vi "Transfer State 3 test.vi"() -> ()   [LabVIEW 2019]
panel:
  out "s? t:f":dbl
  in  "x":bool
  in  "Reset":bool
  in  "Transfer Forward Slow":dbl
  in  "Transfer Rev slow":dbl
  in  "Transfer Rev Fast":dbl
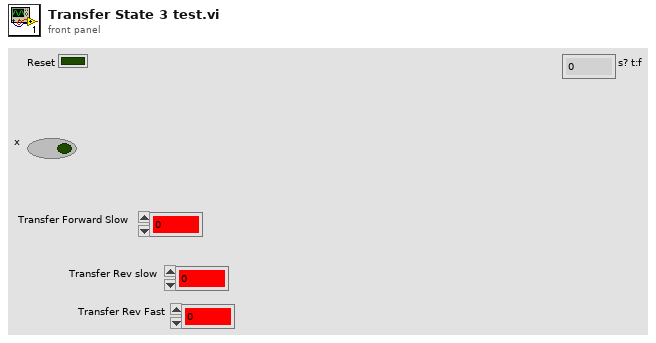
[diagram p1: front panel]
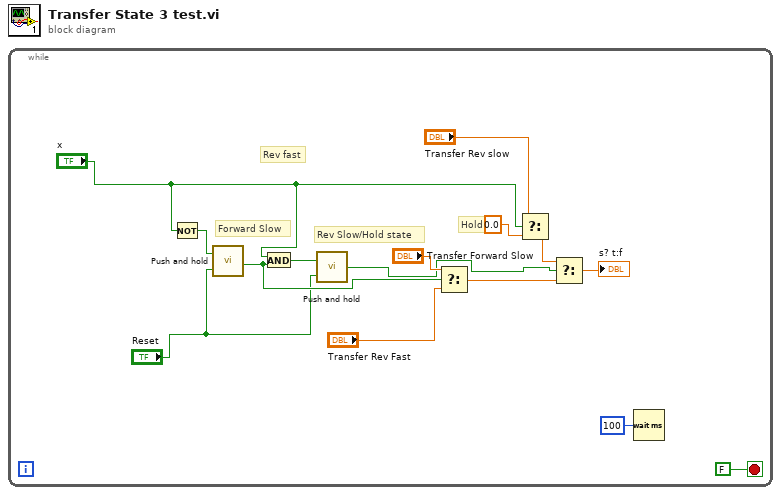
[diagram p0: block diagram]
diagram:
  n1 = while {
    stop <- FALSE stop-if-true
    # "Hold"
    # "Rev Slow/Hold state"
    # "Forward Slow"
    # "Rev fast"
    n2 = Not(x="x") -> (.not. x?=w15:bool)
    n3 = call "Push and hold.vi"("Reset"="Reset", "Input"=w15) -> ("Output"=w12:bool)
    n4 = And(x="x", y=w12) -> (x .and. y?=w14:bool)
    n5 = call "Push and hold.vi"("Reset"="Reset", "Input"=w14) -> ("Output"=w10:bool)
    n6 = Select(t="Transfer Forward Slow", s=w12, f="Transfer Rev Fast") -> (s? t:f=w9:dbl)
    n7 = Select(t="Transfer Rev slow", s="x", f=0.0 ("Setpoint")) -> (s? t:f=w6:dbl)
    n8 = Select(t=w6, s=w10, f=w9) -> (s? t:f=→"s? t:f":dbl)
    n9 = Wait (ms)(milliseconds to wait=u32 100) -> ()  [unwired: 1 out]
  }
